vi "DVR Access.vi"(0 "Stop":bool, 11 "error in":errorcluster) -> (4 "DVR value":dbl, 6 "Loop 1 DVR data":dbl, 8 "Loop 2 Data":dbl, 10 "Loop 3 DVR Data":dbl, 15 "error out":errorcluster)   [LabVIEW 2023]
panel:
  # "INSTRUCTIONS :\n\n1. Run the VI.\n2. Observe the DVR data from different \n    loops running at different wait time.\n3. Press Stop to abort the VI.\n4. Based on the observation, behavior is\n    documented."
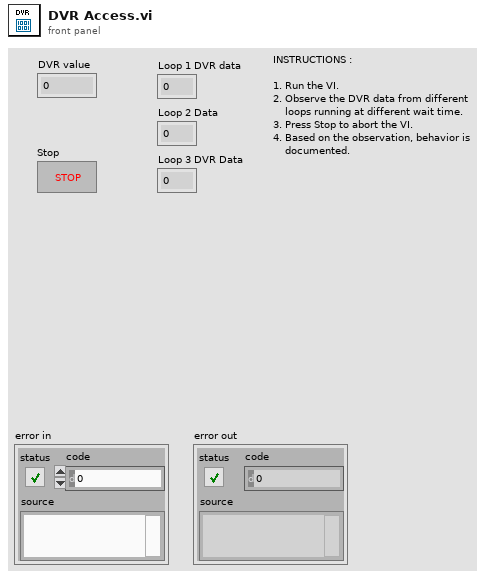
[diagram p1: front panel]
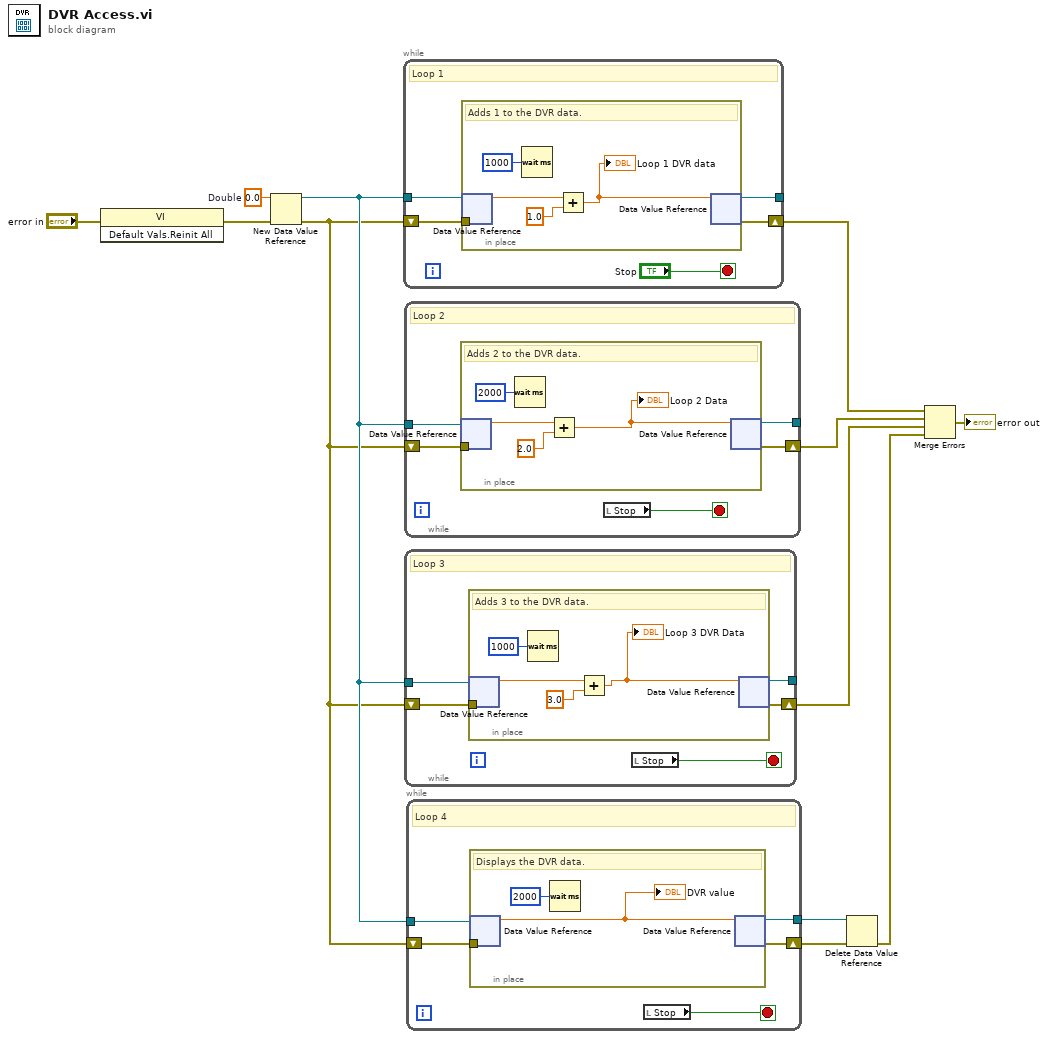
[diagram p0: block diagram]
diagram:
  w12 = 0.0  # Double
  n1 = invoke class="VI" method="Default Vals.Reinit All"(error in="error in") -> (error out=w1:errorcluster)  [unwired: 2 in, 2 out]
  n2 = New Data Value Reference(data value=w12, error in=w1) -> (data value reference=w11:refnum<data-value>, error out=w9:errorcluster)
  n3 = while {
    tunnel: w11 -> [w17]
    tunnel: [w16] -> _
    shift-right: [w14] -> w7
    shift-left: w9 -> [w13]
    stop <- "Stop" stop-if-true
    # "Loop 1"
    n4 = in-place {
      in-place-border: w13 -> [_]
      # "Adds 1 to the DVR data."
      n5 = in-place-dvr #1(w17) -> (w19:dbl)  [unwired: 1 out]
      n6 = Wait (ms)(milliseconds to wait=u32 1000) -> ()  [unwired: 1 out]
      n7 = Add(x=w19, y=1.0) -> (x+y=w21:dbl)
      "Loop 1 DVR data" <- w21
      n8 = in-place-dvr #1(w21) -> (w16:refnum<data-value>, w14:errorcluster)
    }
  }
  n9 = while {
    tunnel: w11 -> [w26]
    tunnel: [w25] -> _
    shift-right: [w22] -> w6
    shift-left: w9 -> [w23]
    stop <- w24 stop-if-true
    # "Loop 2"
    n10 = in-place {
      in-place-border: w23 -> [_]
      # "Adds 2 to the DVR data."
      n11 = in-place-dvr #2(w26) -> (w28:dbl)  [unwired: 1 out]
      n12 = Wait (ms)(milliseconds to wait=u32 2000) -> ()  [unwired: 1 out]
      n13 = Add(x=w28, y=2.0) -> (x+y=w27:dbl)
      "Loop 2 Data" <- w27
      n14 = in-place-dvr #2(w27) -> (w25:refnum<data-value>, w22:errorcluster)
    }
    n15 = local read "Stop"() -> (w24:bool)
  }
  n16 = while {
    tunnel: w11 -> [w35]
    tunnel: [w34] -> _
    shift-right: [w31] -> w5
    shift-left: w9 -> [w32]
    stop <- w33 stop-if-true
    # "Loop 3"
    n17 = in-place {
      in-place-border: w32 -> [_]
      # "Adds 3 to the DVR data."
      n18 = in-place-dvr #3(w35) -> (w37:dbl)  [unwired: 1 out]
      n19 = Wait (ms)(milliseconds to wait=u32 1000) -> ()  [unwired: 1 out]
      n20 = Add(x=w37, y=3.0) -> (x+y=w36:dbl)
      "Loop 3 DVR Data" <- w36
      n21 = in-place-dvr #3(w36) -> (w34:refnum<data-value>, w31:errorcluster)
    }
    n22 = local read "Stop"() -> (w33:bool)
  }
  n23 = while {
    tunnel: w11 -> [w44]
    tunnel: [w43] -> w10
    shift-right: [w40] -> w8
    shift-left: w9 -> [w41]
    stop <- w42 stop-if-true
    # "Loop 4"
    n24 = in-place {
      in-place-border: w41 -> [_]
      # "Displays the DVR data."
      n25 = in-place-dvr #4(w44) -> (w45:dbl)  [unwired: 1 out]
      "DVR value" <- w45
      n26 = Wait (ms)(milliseconds to wait=u32 2000) -> ()  [unwired: 1 out]
      n27 = in-place-dvr #4(w45) -> (w43:refnum<data-value>, w40:errorcluster)
    }
    n28 = local read "Stop"() -> (w42:bool)
  }
  n29 = Delete Data Value Reference(data value reference=w10, error in=w8) -> (error out=w4:errorcluster)  [unwired: 1 out]
  n30 = Merge Errors(w7, w6, w5, w4) -> (→"error out":errorcluster)
